vi "Disconnect.vi"(1 "Fehler (Eingang, kein Fehler)":errorcluster caption="error in", 2 "Com Port in":refnum<visa-resource-name>) -> (0 "Fehler (Ausgang)":errorcluster caption="error out")   [LabVIEW 2013]
doc: "Disconnects a Omicron device from the computer. The COM port is closed."
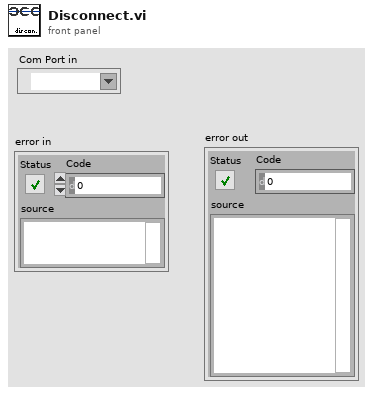
[diagram p1: front panel]
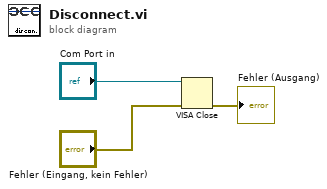
[diagram p0: block diagram]
diagram:
  n1 = VISA Close(VISA resource name="Com Port in", error in (no error)="Fehler (Eingang, kein Fehler)") -> (error out=→"Fehler (Ausgang)":errorcluster)
